vi "configureOutput.vi"(6 "sofwareTrigger?":bool, 8 "error in (no error)":errorcluster, 9 "Data":variant, 10 "Config":T1, 11 "CQT_DDS in":refnum<class "CQT_DDS.lvclass">) -> (0 "error out":errorcluster, 3 "CQT_DDS out":refnum<class "CQT_DDS.lvclass">)   [LabVIEW 2011, in "CQT_DDS.lvclass"]
doc: "Data is an array of varient clusters. One varient cluster per channel.\n\nVariant is a 2D array { {Time, Freq, Amplitude,Phase},...}"
uses:
  CQT_DDS.lvclass
  Generic/DDSOutput.lvclass
  CQT_DDS.lvclass/CQT_DDS.ctl
panel:
  out "data (time, freq, amplitude, phase)":dbl[][](array[numeric]) format="%#.7g"
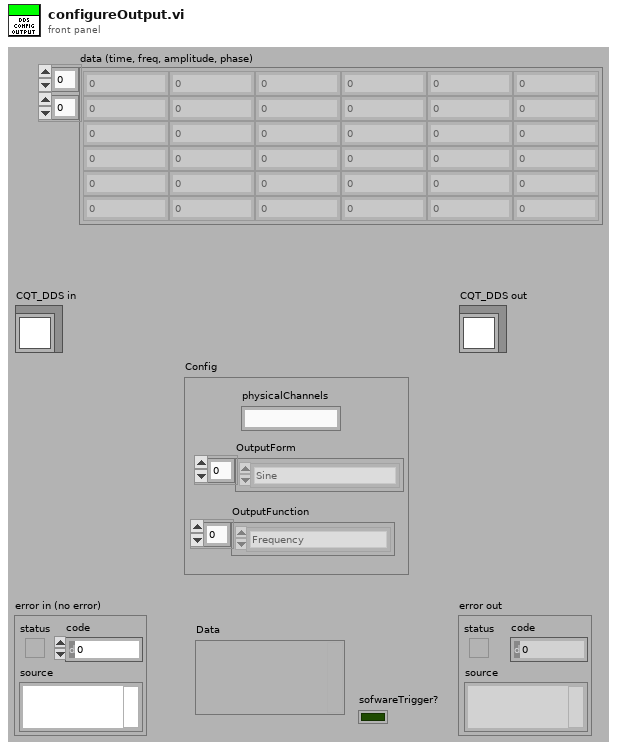
[diagram p1: front panel]
types:
  T1 = cluster{"OutputForm":enum16{"Sine", "Square", "Triangle", "Arbitrary"}[], "OutputFunction":enum16{"Frequency", "Ramp", "Sequence"}[], "physicalChannels":string}
  T2 = cluster{"Frequency(MHz)":dbl, "Amplitude":dbl, "Phase":dbl, "OutputForm":enum16{"Sine", "Square", "Triangle", "Arbitrary"}}[]
  T3 = cluster{"data (time, freq, amplitude, phase)":dbl[][]}
  T4 = cluster{"data (time, freq, amplitude, phase)":dbl[][]}[]
  T5 = cluster{"Frequency(MHz)":dbl, "Amplitude":dbl, "Phase":dbl, "OutputForm":enum16{"Sine", "Square", "Triangle", "Arbitrary"}}
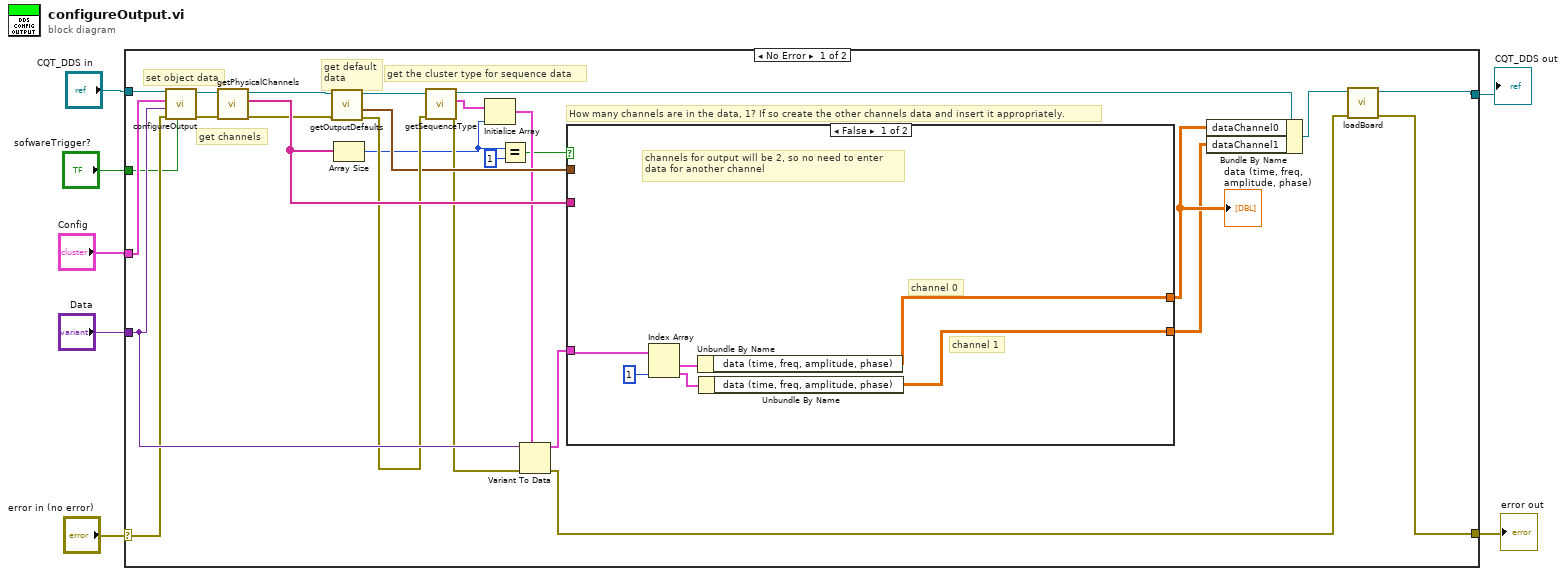
[diagram p0: block diagram]
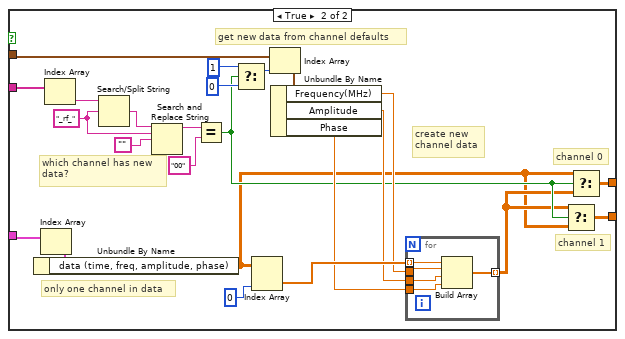
[diagram p2: hidden frame]
diagram:
  n1 = case shown="No Error" "error in (no error)" {
    selector: "error in (no error)" -> [w15 w70]
    tunnel: [w8 w70] -> w2
    tunnel: [w10 w71] -> w3
    tunnel: "CQT_DDS in" -> [w34 w71]
    tunnel: "Config" -> [w33 _]
    tunnel: "Data" -> [w29 _]
    tunnel: "sofwareTrigger?" -> [w12 _]
    frame No Error {
      # "get default\ndata"
      # "get channels"
      # "set object data"
      # "get the cluster type for sequence data"
      # "How many channels are in the data, 1? If so create the other channels data and insert it appropriately."
      n2 = call-parent "configureOutput.vi"("sofwareTrigger?"=w12, "error in (no error)"=w15, "Data"=w29, "Config"=w33, "DDSOutput in"=w34) -> ("error out"=w32:errorcluster, "DDSOutput out"=w31:refnum<class "CQT_DDS.lvclass">)  [unwired: 5 in]
      n3 = call "getPhysicalChannels.vi"("error in (no error)"=w32, "DDSOutput in"=w31) -> ("error out"=w27:errorcluster, "physicalChannels"=w30:string[], "DDSOutput out"=w14:refnum<class "CQT_DDS.lvclass">)  [unwired: 7 in]
      n4 = call "getOutputDefaults.vi"("error in (no error)"=w27, "DDSOutput in"=w14) -> ("error out"=w26:errorcluster, "Defaults"=w25:T2, "DDSOutput out"=w28:refnum<class "CQT_DDS.lvclass">)  [unwired: 6 in, 1 out]
      n5 = Array Size(array=w30) -> (size(s)=w18:i32)
      n6 = call "getSequenceType.vi"("error in (no error)"=w26, "DDSOutput in"=w28) -> ("error out"=w23:errorcluster, "Sequence"=w24:T3, "DDSOutput out"=w21:refnum<class "CQT_DDS.lvclass">)  [unwired: 7 in]
      n7 = Initialize Array(w24, w18) -> (w22:T4)
      n8 = Equal?(x=w18, y=1) -> (x = y?=w17:bool)
      n9 = Variant To Data(error in=w23, type=w22, Variant=w29) -> (data=w20:T4, error out=w9:errorcluster)
      n10 = case shown="False" w17 {
        tunnel: w30 -> [_ w60]
        tunnel: w25 -> [_ w53]
        tunnel: w20 -> [w40 w54]
        tunnel: [w38 w44] -> w19
        tunnel: [w36 w43] -> w13
        frame False {
          # "channel 1"
          # "channel 0"
          # "channels for output will be 2, so no need to enter\ndata for another channel"
          n11 = Index Array(array=w40, index #2=1) -> (element #1=w39:T3, element #2=w37:T3)  [unwired: 1 in]
          n12 = Unbundle By Name(w39) -> ("data (time, freq, amplitude, phase)"=w38:dbl[][])
          n13 = Unbundle By Name(w37) -> ("data (time, freq, amplitude, phase)"=w36:dbl[][])
        }
        frame True {
          w62 = "_rf_"
          # "get new data from channel defaults"
          # "only one channel in data"
          # "create new\nchannel data"
          # "channel 1"
          # "channel 0"
          # "which channel has new\ndata?"
          n14 = Index Array(array=w54) -> (element=w52:T3)  [unwired: 1 in]
          n15 = Unbundle By Name(w52) -> ("data (time, freq, amplitude, phase)"=w41:dbl[][])
          n16 = Index Array(array=w60) -> (element=w64:string)  [unwired: 1 in]
          n17 = Search/Split String(string=w64, search string/char (-)=w62) -> (match + rest of string=w63:string)  [unwired: 1 in, 2 out]
          n18 = Search and Replace String(input string=w63, search string=w62, replace string="") -> (result string=w58:string)  [unwired: 5 in, 3 out]
          n19 = Equal?(x=w58, y="00") -> (x = y?=w45:bool)
          n20 = Select(t=1, s=w45, f=0) -> (s? t:f=w57:i32)
          n21 = Index Array(array=w41, index (col)=0) -> (element=w49:dbl[])  [unwired: 1 in]
          n22 = Index Array(array=w53, index=w57) -> (element=w51:T5)
          n23 = Unbundle By Name(w51) -> ("Frequency(MHz)"=w48:dbl, "Amplitude"=w47:dbl, "Phase"=w46:dbl)
          n24 = for {
            tunnel: w49 -> [w69] mode=indexing
            tunnel: w48 -> [w68]
            tunnel: w47 -> [w67]
            tunnel: w46 -> [w66]
            tunnel: [w65] -> w42 mode=indexing
            n25 = Build Array(w69, w68, w67, w66) -> (w65:dbl[])
          }
          n26 = Select(t=w42, s=w45, f=w41) -> (s? t:f=w43:dbl[][])
          n27 = Select(t=w41, s=w45, f=w42) -> (s? t:f=w44:dbl[][])
        }
      }
      "data (time, freq, amplitude, phase)" <- w19
      n28 = Bundle By Name(cluster=w21, "dataChannel0"=w19, "dataChannel1"=w13) -> (w11:refnum<class "CQT_DDS.lvclass">)
      n29 = call "loadBoard.vi"("error in (no error)"=w9, "CQT_DDS in"=w11) -> ("error out"=w8:errorcluster, "CQT_DDS out"=w10:refnum<class "CQT_DDS.lvclass">)  [unwired: 8 in]
    }
    frame Error {
    }
  }
  "error out" <- w2
  "CQT_DDS out" <- w3
